vi "Write States.vi"(8 "error in (no error)":errorcluster, 10 "States":T1=enum."GoToReceiveTable", 11 "KickToPassReceiverTactic in":refnum<class "KickToPassReceiverTactic.lvclass">) -> (0 "error out":errorcluster, 3 "KickToPassReceiverTactic out":refnum<class "KickToPassReceiverTactic.lvclass">)   [LabVIEW 2021, in "KickToPassReceiverTactic.lvclass"]
uses:
  KickToPassReceiverTactic.lvclass
  KickToPassReceiverTacticStates.ctl
  KickToPassReceiverTactic.lvclass/KickToPassReceiverTactic.ctl
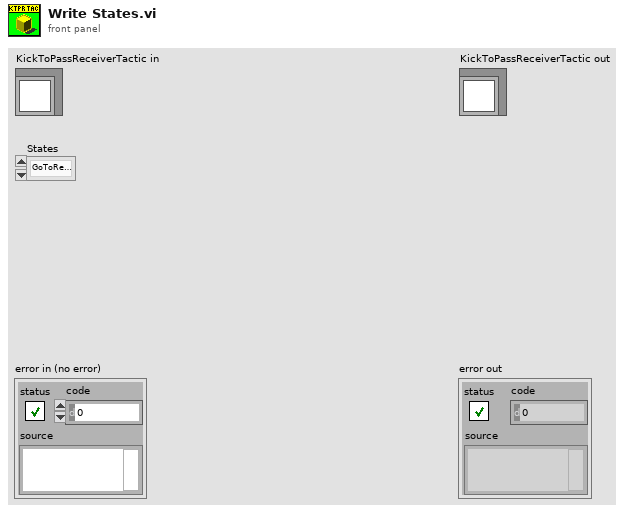
[diagram p1: front panel]
types:
  T1 = typedef "KickToPassReceiverTacticStates.ctl" = enum16{"Halt", "GoToReceiveTable", "KickToPassReceiver", "WaitPass", "Exit"}
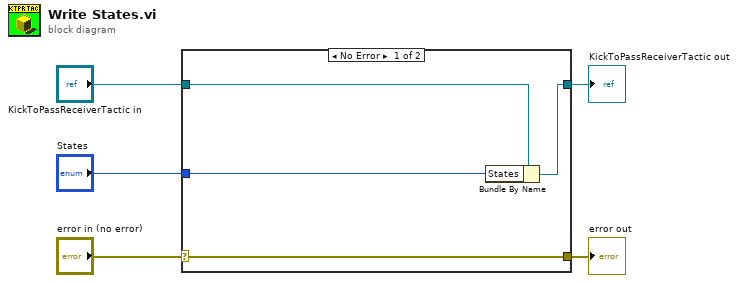
[diagram p0: block diagram]
diagram:
  n1 = case shown="No Error" "error in (no error)" {
    selector: "error in (no error)" -> [w9 w10]
    tunnel: [w9 w10] -> w4
    tunnel: [w7 w11] -> w2
    tunnel: "KickToPassReceiverTactic in" -> [w8 w11]
    tunnel: "States" -> [w6 _]
    frame No Error {
      n2 = Bundle By Name(cluster=w8, "States"=w6) -> (w7:refnum<class "KickToPassReceiverTactic.lvclass">)
    }
    frame Error {
    }
  }
  "error out" <- w4
  "KickToPassReceiverTactic out" <- w2
